vi "Query Configuration List.vi"(0 "VISA resource name":refnum<visa-resource-name>, 5 "List Name":string="MyMeasList", 9 "Point":i32, 11 "error in (no error)":errorcluster) -> (4 "VISA resource name out":refnum<visa-resource-name>, 6 "TSP commands List":string, 15 "error Out (no error)":errorcluster)   [LabVIEW 2016, in "Keithley DMM7510.lvlib"]
doc: "This VI returns a list of TSP commands that represent the parameters that are stored in the specified configuration point."
uses:
  Keithley DMM7510.lvlib
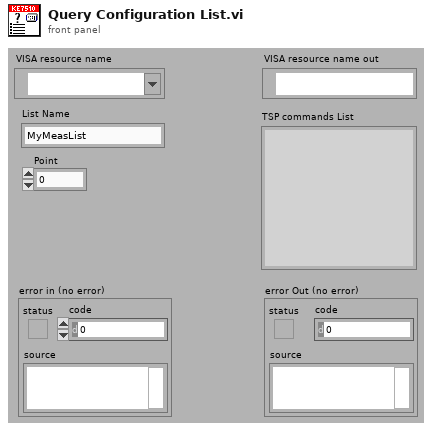
[diagram p1: front panel]
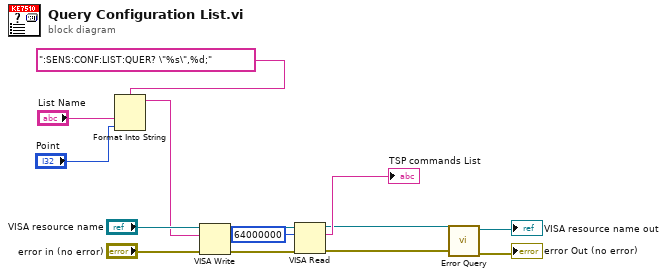
[diagram p0: block diagram]
diagram:
  n1 = Format Into String(format string=":SENS:CONF:LIST:QUER? \"%s\",%d;", "List Name", "Point") -> (resulting string=w11:string)  [unwired: 2 in, 1 out]
  n2 = VISA Write(VISA resource name="VISA resource name", write buffer=w11, error in (no error)="error in (no error)") -> (VISA resource name out=w6:refnum<visa-resource-name>, error out=w5:errorcluster)  [unwired: 1 out]
  n3 = VISA Read(VISA resource name=w6, byte count=u32 64000000, error in (no error)=w5) -> (VISA resource name out=w2:refnum<visa-resource-name>, read buffer=→"TSP commands List":string, error out=w1:errorcluster)  [unwired: 1 out]
  n4 = call "Error Query.vi"("error in (no error)"=w1, "VISA resource name"=w2) -> ("error out"=→"error Out (no error)":errorcluster, "VISA resource name out"=→"VISA resource name out":refnum<visa-resource-name>)  [unwired: 6 in, 2 out]
